vi "Register For Events.vi"(8 "error in":errorcluster, 11 "lia rt in":refnum<class "Lock-In Amplifier Example RT.lvclass">) -> (0 "error out":errorcluster, 2 "event":refnum<event-registration>, 3 "lia rt out":refnum<class "Lock-In Amplifier Example RT.lvclass">)   [LabVIEW 2017, in "Lock-In Amplifier Example RT.lvclass"]
uses:
  Lock-In Amplifier Example RT.lvclass
  server/Public/State.ctl
  Properties/Server_GET.vi
  server/Properties/StateChangedEvent_GET.vi
  server/RT FlexRIO Server TCP.lvclass
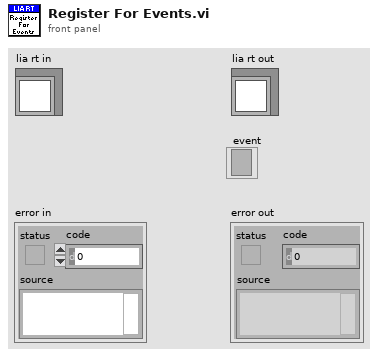
[diagram p1: front panel]
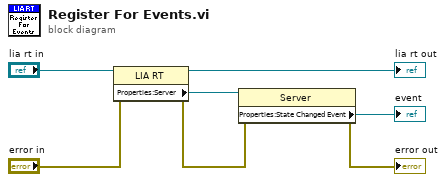
[diagram p0: block diagram]
diagram:
  n1 = property class="LIA RT"(reference="lia rt in", error in="error in") -> (reference out=→"lia rt out":refnum<class "Lock-In Amplifier Example RT.lvclass">, error out=w3:errorcluster, "Properties:Server"=w4:refnum<class "RT FlexRIO Server TCP.lvclass">)
  n2 = property class="Server"(reference=w4, error in=w3) -> (error out=→"error out":errorcluster, "Properties:State Changed Event"=→"event":refnum<event-registration>)  [unwired: 1 out]
